vi "createTableCells.vi"(8 "error in (no error)":errorcluster, 10 "Table":string[][](array[string]), 11 "Table Ref in":refnum<k24>) -> (0 "error out":errorcluster, 3 "Table Ref out":refnum<k24>)   [LabVIEW 2017, in "LabVIEW NPOI.lvlib" / "MS-Word.lvclass"]
uses:
  MS-Word.lvclass
  C:/Users/Neo/Desktop/Dev_Tools_BR/LabVIEW_NPOI/lib/NPOI 2.1.1/NPOI.OOXML.dll
  lib/NPOI 2.1.1/NPOI.OOXML.dll
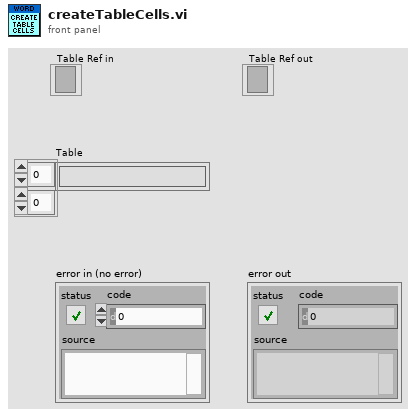
[diagram p1: front panel]
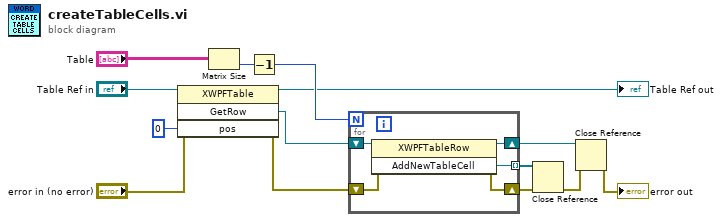
[diagram p0: block diagram]
diagram:
  n1 = invoke class="XWPFTable" method="GetRow"(reference="Table Ref in", error in="error in (no error)", "pos"=0) -> (reference out=→"Table Ref out":refnum<k24>, error out=w6:errorcluster, "GetRow"=w12:refnum<k24>)  [unwired: 1 in, 1 out]
  n2 = Matrix Size(0:"Table") -> (2:w13:i32)  [unwired: 1 out]
  n3 = Decrement(x=w13) -> (x-1=w11:i32)
  n4 = for {
    N: w11 -> [_]
    shift-right: [w18] -> w7
    shift-left: w12 -> [w19]
    tunnel: [w17] -> w9 mode=indexing
    shift-right: [w16] -> w10
    shift-left: w6 -> [w15]
    n5 = invoke class="XWPFTableRow" method="AddNewTableCell"(reference=w19, error in=w15) -> (reference out=w18:refnum<k24>, error out=w16:errorcluster, "AddNewTableCell"=w17:refnum<k24>)  [unwired: 1 in]
  }
  n6 = Close Reference(reference=w9, error in (no error)=w10) -> (error out=w8:errorcluster)
  n7 = Close Reference(reference=w7, error in (no error)=w8) -> (error out=→"error out":errorcluster)
